vi "ONOFFcontrol.vi"(11 "Output ON/OFF (T: ON)":bool) -> (0 "error out":errorcluster)   [LabVIEW 2024]
uses:
  old LabVIEW files/labview_Mikami/Teledyne LeCroy WaveStation/Teledyne LeCroy WaveStation.lvlib
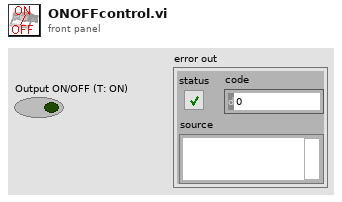
[diagram p1: front panel]
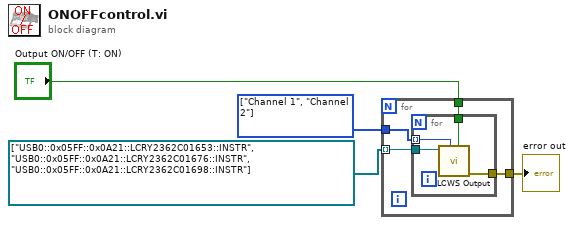
[diagram p0: block diagram]
diagram:
  w3 = enum16{"Channel 1", "Channel 2"}[] [enum."Channel 1", enum."Channel 2"] items=["Channel 1", "Channel 2"]
  n1 = for {
    tunnel: refnum<visa-resource-name>[] ["USB0::0x05FF::0x0A21::LCRY2362C01653::INSTR", "USB0::0x05FF::0x0A21::LCRY2362C01676::INSTR", "USB0::0x05FF::0x0A21::LCRY2362C01698::INSTR"] -> [w8] mode=indexing
    tunnel: w3 -> [w7]
    tunnel: "Output ON/OFF (T: ON)" -> [w6]
    tunnel: [w5] -> w1
    n2 = for {
      tunnel: w8 -> [w12]
      tunnel: w7 -> [w11] mode=indexing
      tunnel: w6 -> [w10]
      tunnel: [w9] -> w5
      n3 = call "LCWS Output.vi"("Output ON/OFF (T: ON)"=w10, "Channel (1)"=w11, "VISA resource name"=w12) -> ("error out"=w9:errorcluster)  [unwired: 7 in, 1 out]
    }
  }
  "error out" <- w1
